vi "EXAMPLE APPLICATION.vi"() -> ()   [LabVIEW 2021]
uses:
  <vilib>/Instr/_visa.llb/VISA Configure Serial Port (Instr).vi
panel:
  in  "EMERGENCY":bool
  in  "Slide":u8(slide) scale=0.0..255.0
  out "Slide MCU Response":dbl(knob) scale=0.0..255.0
  out "Written?":bool
  out "Data to Send":i32[](array[numeric])
  out "(hi.lo)":u16
  out "Potentiometer:":dbl(knob) scale=0.0..1023.0
  in  "Start":bool
  in  "Write?":bool
  out "DBarray":dbl[][](array[numeric])
  in  "DB File":string="cansart_db.h"
  in  "stop":bool
  in  "BaudRate:":u32=115200
  in  "COM:":refnum<visa-resource-name>
  # "Cansart Example Application"
  # "Test Potentiometer by connecting a potentiometer\non the pin referred on your controller example"
  # "Double Click on the 1023 number to change it \nto a higher number depending on what your \nADC resolution"
  # "Engineered and Maintained by:\nGuilherme Candido\nteoriaeletrica@gmail.com"
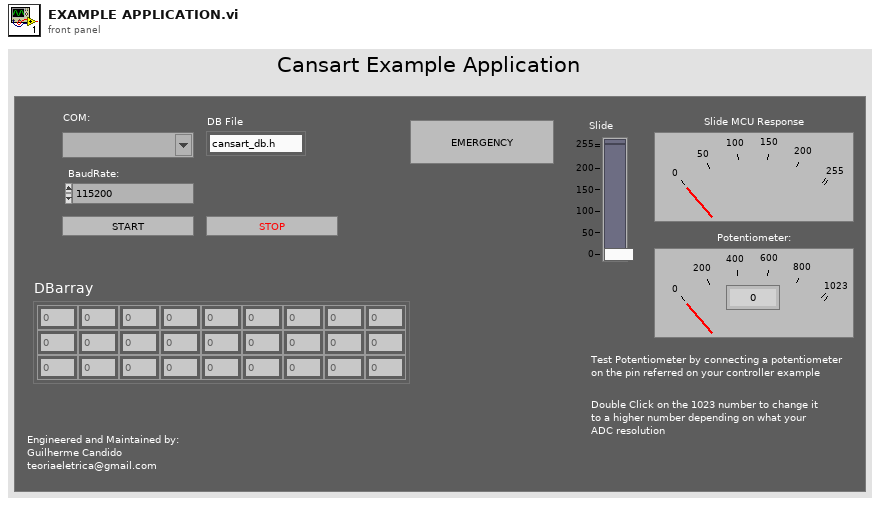
[diagram p1: front panel]
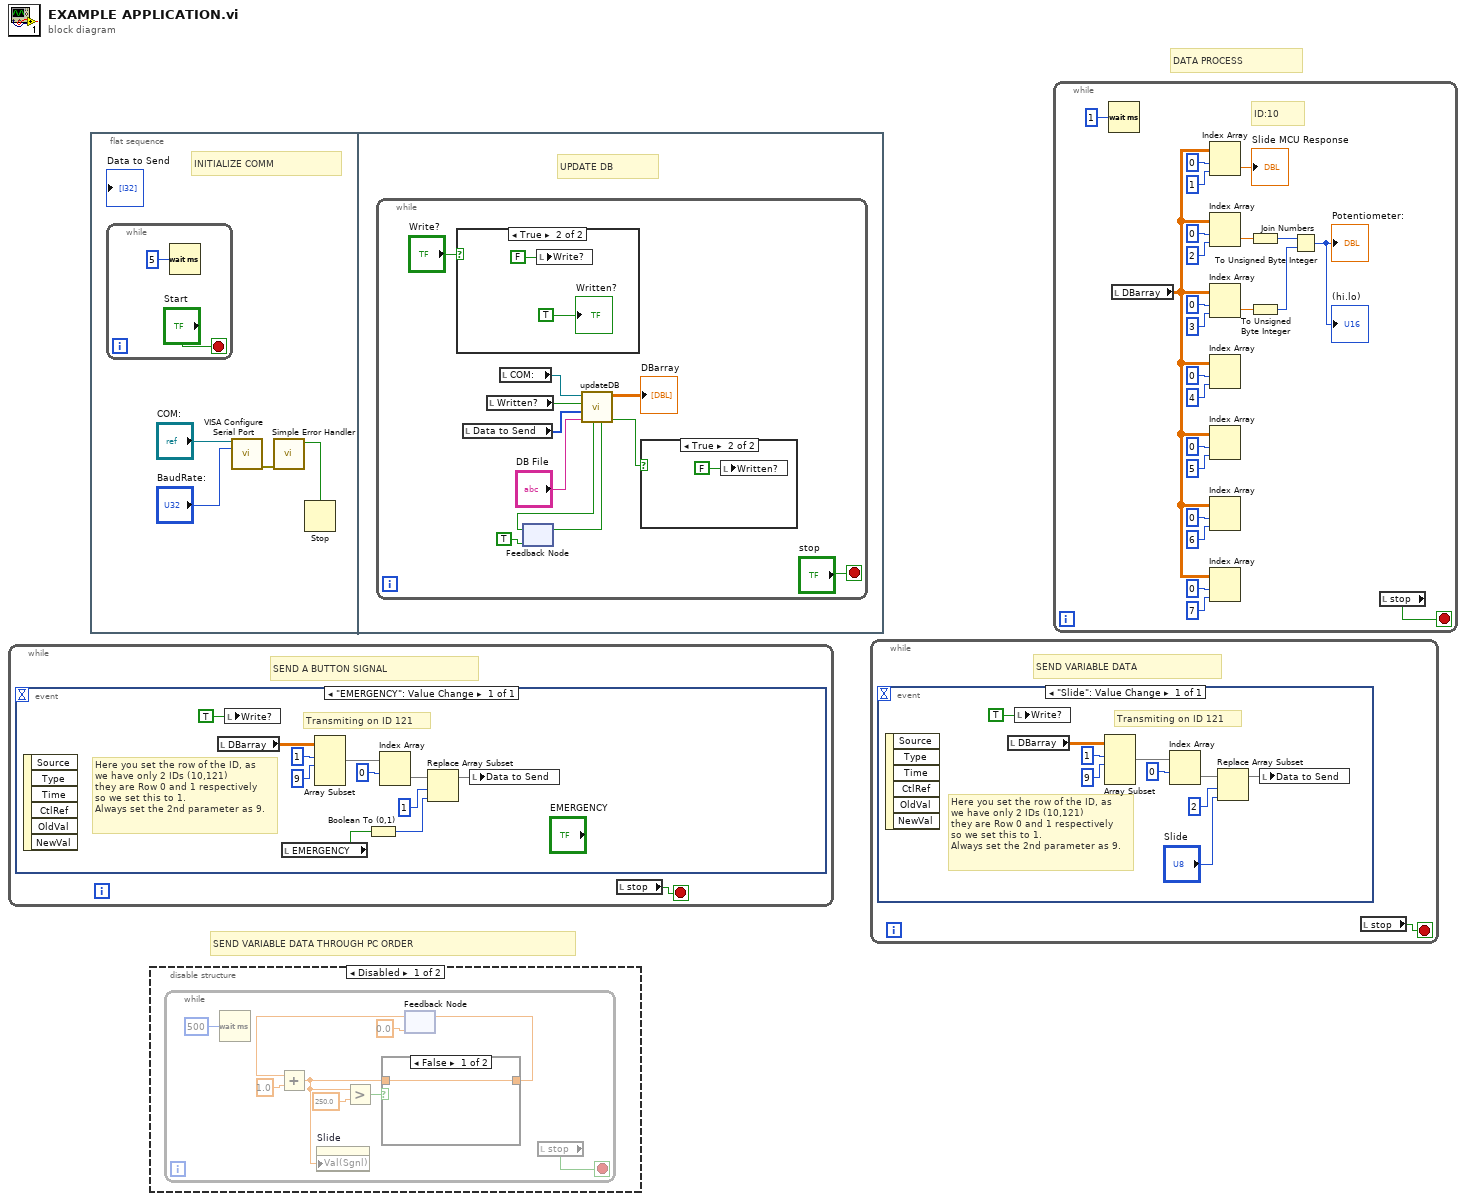
[diagram p0: block diagram]
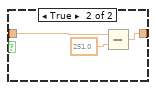
[diagram p2: hidden frame]
diagram:
  # "DATA PROCESS"
  # "SEND VARIABLE DATA THROUGH PC ORDER"
  n1 = while {
    stop <- w1 stop-if-true
    # "SEND A BUTTON SIGNAL"
    n2 = event shown="[0] \"EMERGENCY\": Value Change" {
      selector: _ -> [_]
      dyn-events: _ -> [_]
      timeout: _ -> [_]
      event "EMERGENCY": Value Change {
        # "Here you set the row of the ID, as \nwe have only 2 IDs (10,121) \nthey are Row 0 and 1 respectively \nso we set this to 1.\nAlways set the 2nd parameter as 9."
        # "Transmiting on ID 121"
        n3 = event-data() -> ()  [unwired: 1 in, 6 out]
        n4 = local read "DBarray"() -> (w8:dbl[][])
        n5 = local write "Write?"(TRUE ("Write?")) -> ()
        n6 = local read "EMERGENCY"() -> (w11:bool)
        n7 = Array Subset(array=w8, index (row)=1 ("index"), length (row)=9 ("length")) -> (w7:dbl[][])  [unwired: 2 in]
        n8 = Boolean To (0,1)(Boolean=w11) -> (0, 1=w2:i16)
        n9 = Index Array(array=w7, index (row)=0) -> (element=w9:dbl[])  [unwired: 1 in]
        n10 = Replace Array Subset(array=w9, new element=w2, index=1) -> (w10:dbl[])
        n11 = local write "Data to Send"(w10) -> ()
      }
    }
    n12 = local read "stop"() -> (w1:bool)
  }
  n13 = flat-sequence {
    frame #0 {
      # "INITIALIZE COMM"
      n14 = while {
        stop <- "Start" stop-if-true
        n15 = Wait (ms)(milliseconds to wait=u32 5) -> ()  [unwired: 1 out]
      }
      n16 = call-poly "VISA Configure Serial Port"("VISA resource name"="COM:", "baud rate (9600)"="BaudRate:") -> ("error out"=w14:errorcluster)  [unwired: 12 in, 1 out]
      n17 = call <vilib>:"Simple Error Handler.vi"("error in (no error)"=w14) -> ("error?"=w13:bool)  [unwired: 4 in, 4 out]
      n18 = Stop(stop? (T)=w13) -> ()
    }
    frame #1 {
      # "UPDATE DB"
      n19 = while {
        stop <- "stop" stop-if-true
        n20 = case shown="True" "Write?" {
          frame False {
          }
          frame True {
            n21 = local write "Write?"(FALSE ("Write?")) -> ()
            "Written?" <- TRUE ("Boolean")
          }
        }
        n22 = local read "Data to Send"() -> (w24:i32[])
        n23 = local read "Written?"() -> (w21:bool)
        n24 = local read "COM:"() -> (w28:refnum<visa-resource-name>)
        n25 = feedback #1(TRUE ("First 2")) -> (w20:bool)
        n26 = call "updateDB.vi"("First"=w20, "DBname"="DB File", "Data Write"=w24, "Write?"=w21, "COM PORT"=w28) -> ("Written!"=w22:bool, "DBarray"=→"DBarray":dbl[][], "First 2"=w19:bool)  [unwired: 4 in]
        n27 = feedback-in #1(w19) -> ()
        n28 = case shown="True" w22 {
          frame False {
          }
          frame True {
            n29 = local write "Written?"(FALSE ("Written?")) -> ()
          }
        }
      }
    }
  }
  n30 = disable-structure shown="Disabled" {
    frame Disabled {
      n31 = while {
        stop <- w41 stop-if-true
        n32 = Wait (ms)(milliseconds to wait=u32 500) -> ()  [unwired: 1 out]
        n33 = feedback #2(0.0) -> (w35:dbl)
        n34 = Add(x=w35, y=1.0) -> (x+y=w33:dbl)
        n35 = property on="Slide" class="Slide (strict)"("Val(Sgnl)"=w33) -> ()  [unwired: 2 in, 2 out]
        n36 = Greater?(x=w33, y=250.0) -> (0:w37:bool)
        n37 = case shown="False" w37 {
          tunnel: [w42 w44] -> w36
          tunnel: w33 -> [w42 w43]
          frame False {
          }
          frame True {
            n38 = Subtract(x=w43, y=251.0) -> (x-y=w44:dbl)
          }
        }
        n39 = feedback-in #2(w36) -> ()
        n40 = local read "stop"() -> (w41:bool)
      }
    }
    frame Enabled {
    }
  }
  n41 = while {
    stop <- w46 stop-if-true
    # "SEND VARIABLE DATA"
    n42 = event shown="[0] \"Slide\": Value Change" {
      selector: _ -> [_]
      dyn-events: _ -> [_]
      timeout: _ -> [_]
      event "Slide": Value Change {
        # "Here you set the row of the ID, as \nwe have only 2 IDs (10,121) \nthey are Row 0 and 1 respectively \nso we set this to 1.\nAlways set the 2nd parameter as 9."
        # "Transmiting on ID 121"
        n43 = event-data() -> ()  [unwired: 1 in, 6 out]
        n44 = local read "DBarray"() -> (w50:dbl[][])
        n45 = local write "Write?"(TRUE ("Write?")) -> ()
        n46 = Array Subset(array=w50, index (row)=1 ("index"), length (row)=9 ("length")) -> (w55:dbl[][])  [unwired: 2 in]
        n47 = Index Array(array=w55, index (row)=0) -> (element=w56:dbl[])  [unwired: 1 in]
        n48 = Replace Array Subset(array=w56, new element="Slide", index=2) -> (w48:dbl[])
        n49 = local write "Data to Send"(w48) -> ()
      }
    }
    n50 = local read "stop"() -> (w46:bool)
  }
  n51 = while {
    stop <- w69 stop-if-true
    # "ID:10"
    n52 = Wait (ms)(milliseconds to wait=u32 1) -> ()  [unwired: 1 out]
    n53 = local read "DBarray"() -> (w63:dbl[][])
    n54 = Index Array(array=w63, index (row)=0, index (col)=1 ("disabled index (col)")) -> (element=→"Slide MCU Response":dbl)
    n55 = Index Array(array=w63, index (row)=0 ("disabled index (row)"), index (col)=2 ("disabled index (col)")) -> (element=w75:dbl)
    n56 = Index Array(array=w63, index (row)=0 ("disabled index (row)"), index (col)=3 ("disabled index (col)")) -> (element=w78:dbl)
    n57 = Index Array(array=w63, index (row)=0 ("disabled index (row)"), index (col)=4 ("disabled index (col)")) -> ()  [unwired: 1 out]
    n58 = Index Array(array=w63, index (row)=0 ("disabled index (row)"), index (col)=5 ("disabled index (col)")) -> ()  [unwired: 1 out]
    n59 = Index Array(array=w63, index (row)=0 ("disabled index (row)"), index (col)=6 ("disabled index (col)")) -> ()  [unwired: 1 out]
    n60 = Index Array(array=w63, index (row)=0 ("disabled index (row)"), index (col)=7 ("disabled index (col)")) -> ()  [unwired: 1 out]
    n61 = To Unsigned Byte Integer(number=w75) -> (unsigned 8bit integer=w79:u8)
    n62 = To Unsigned Byte Integer(number=w78) -> (unsigned 8bit integer=w77:u8)
    n63 = Join Numbers(hi=w79, lo=w77) -> ((hi.lo)=→"(hi.lo)" →"Potentiometer:":u16)
    n64 = local read "stop"() -> (w69:bool)
  }
